vi "send queue.vi"(6 "zerowanie predkosci":T1[](array[typedef]) {"type" items=["CAN Data", "CAN Remote"]; "identifier" format="%.0x"}, 8 "error in (no error)":errorcluster, 11 "Queue in":refnum<queue>) -> (0 "error out":errorcluster, 3 "queue out":refnum<queue>)   [LabVIEW 2014]
uses:
  CANFrameControl.ctl
  Program Files (x86)/National Instruments/LabVIEW 2014/examples/Design Patterns/Queued Message Handler/support/QMH Fundamentals - Message Cluster.ctl
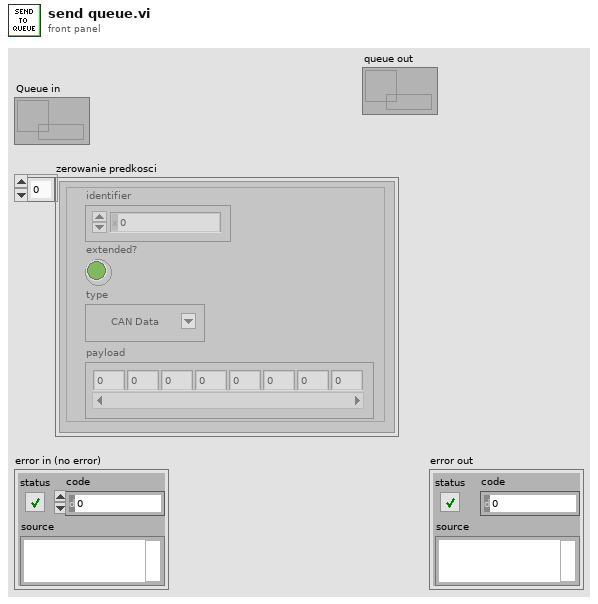
[diagram p1: front panel]
types:
  T1 = typedef "CANFrameControl.ctl" = cluster{"identifier":u32, "extended?":bool, "type":u8, "payload":u8[]}
  T2 = typedef "QMH Fundamentals - Message Cluster.ctl" = cluster{"Message":string, "Message Data":variant}
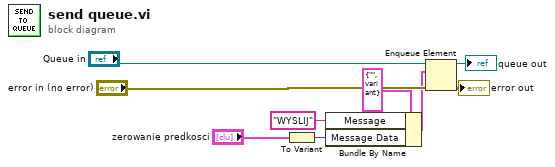
[diagram p0: block diagram]
diagram:
  n1 = To Variant(anything="zerowanie predkosci") -> (Variant=w3:variant)
  n2 = Bundle By Name(cluster=T2 {"Message"="", "Message Data"=variant} ("Message Cluster"), "Message"="WYSLIJ", "Message Data"=w3) -> (w2:T2)
  n3 = Enqueue Element(queue="Queue in", element=w2, error in (no error)="error in (no error)") -> (queue out=→"queue out":refnum<queue>, error out=→"error out":errorcluster)  [unwired: 1 in, 1 out]
